vi "lwr_main.vi"(6 "inputValid":bool, 7 "readAddress":u16, 8 "endOfWave":bool, 9 "startRecording":bool, 10 "satCntP2":u16=12, 11 "input":cluster{"index":u16, "data":i16}) -> (0 "recordReady":bool, 2 "readData":i32, 3 "waveCount":u16)   [LabVIEW 2016]
uses:
  <vilib>/rvi/Emulation/niFpgaEmulationIsFPGAContextNoSignature.vi
  <vilib>/rvi/DataTransferAndStorage/Container/Common/niFpgaContainerGetUniqueNameForEmu.vi
  <vilib>/rvi/Memory/Memory_Emulation/niFpgaMemoryEmulationCacheClearOnFirstRun.vi
  <vilib>/rvi/Memory/Memory_Emulation/nirvimemoryEmulationManagerCache_MakeExclusive.vi
  <vilib>/rvi/Memory/Memory_Emulation/niFpgaMemoryEmulationValidateCache.vi
  <vilib>/rvi/Memory/Memory_Emulation/nirvimemoryEmulationManagerCache_InsertValue.vi
  <vilib>/Utility/error.llb/Clear Errors.vi
  <vilib>/rvi/Memory/Memory_Emulation/nirvimemoryEmulationManagerCache_ReleaseExclusive.vi
  <vilib>/rvi/Memory/Memory_Emulation/nirvimemoryEmulationManagerCache_GetValue.vi
  <vilib>/rvi/Memory/Memory_Emulation/nirvimemoryEmulationManagerCache_SetValue.vi
  <vilib>/rvi/Emulation/niFpgaProcessEmulError.vi
  <vilib>/rvi/Emulation/niFpgaSctlEmulationGetInTimedLoop.vi
  <vilib>/rvi/Memory/Memory_Emulation/nirvimemoryFastEmulation.vi
  <vilib>/rvi/Memory/Memory_Emulation/nirvimemoryEmulation.vi
  <vilib>/rvi/errors/nirviReportUnexpectedCaseInternalError (U32).vi
  <vilib>/rvi/DataTransferAndStorage/Container/XNode/niFpgaContainer.xnode
  <vilib>/rvi/DataTransferAndStorage/Register/Emulation/niFpgaRegisterEmulation.vi
  <instrlib>/_niInstr/Basic Elements/v1/FPGA/niInstr Basic Elements v1 FPGA.lvlib
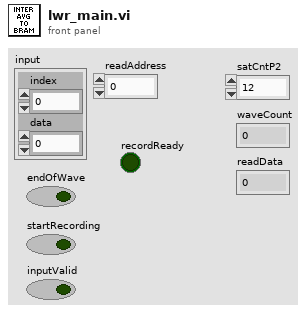
[diagram p1: front panel]
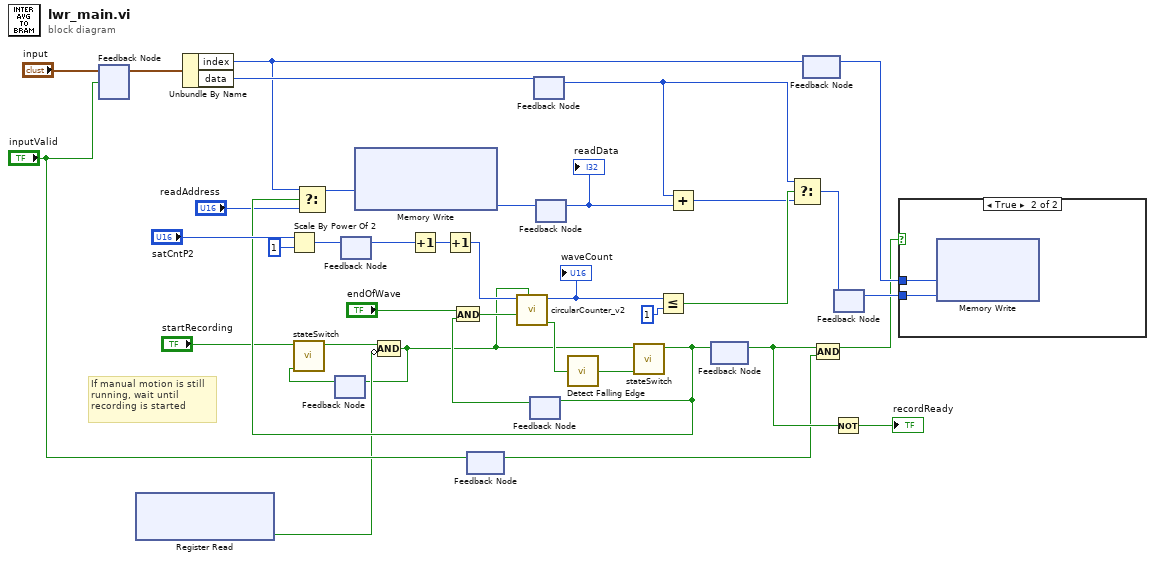
[diagram p0: block diagram]
diagram:
  # "If manual motion is still\nrunning, wait until \nrecording is started"
  n1 = feedback-in #1("input", "inputValid") -> ()
  n2 = feedback #1() -> (w12:cluster{"index":u16, "data":i16})  [unwired: 1 in]
  n3 = xnode ("Register Read")() -> ("Data"=w2:bool)  [unwired: 1 in, 1 out]
  n4 = Unbundle By Name(w12) -> ("index"=w14:u16, "data"=w38:i16)
  n5 = Scale By Power Of 2(n="satCntP2", x=u16 1) -> (x*2^n=w30:u16)
  n6 = feedback #2() -> (w3:bool)  [unwired: 1 in]
  n7 = call "stateSwitch.vi"("disable"=w3, "enable"="startRecording") -> ("state"=w4:bool)  [unwired: 9 in]
  n8 = feedback #3() -> (w34:u16)  [unwired: 1 in]
  n9 = feedback-in #3(w30) -> ()
  n10 = Compound Arithmetic op=AND(w4, invert w2) -> (w1:bool)
  n11 = feedback-in #2(w1) -> ()
  n12 = Increment(x=w34) -> (x+1=w18:u16)
  n13 = Increment(x=w18) -> (x+1=w22:u16)
  n14 = feedback-in #4("inputValid") -> ()
  n15 = feedback #4() -> (w9:bool)  [unwired: 1 in]
  n16 = feedback #5() -> (w24:bool)  [unwired: 1 in]
  n17 = And(x="endOfWave", y=w24) -> (x .and. y?=w37:bool)
  n18 = call "circularCounter_v2.vi"("reset"=w1, "doStep"=w37, "maxCount"=w22) -> ("maxReached"=w25:bool, "index"=w21:u16)  [unwired: 5 in, 2 out]
  "waveCount" <- w21
  n19 = feedback #6() -> (w16:i16)  [unwired: 1 in]
  n20 = feedback-in #6(w38) -> ()
  n21 = feedback #7() -> (w28:i32)  [unwired: 1 in]
  "readData" <- w28
  n22 = call <instrlib>:"Detect Falling Edge.vi"("signal"=w25) -> ("edge detected"=w19:bool)  [unwired: 14 in]
  n23 = call "stateSwitch.vi"("disable"=w19, "enable"=w1) -> ("state"=w7:bool)  [unwired: 9 in]
  n24 = Select(t=w14, s=w7, f="readAddress") -> (s? t:f=w8:u16)
  n25 = xnode ("Memory Write")("Address"=w8) -> ("Data"=w32:i32)  [unwired: 1 in, 1 out]
  n26 = feedback-in #5(w7) -> ()
  n27 = feedback-in #7(w32) -> ()
  n28 = Less Or Equal?(x=w21, y=u16 1) -> (x <= y?=w36:bool)
  n29 = Add(x=w16, y=w28) -> (x+y=w26:i32)
  n30 = feedback #8() -> (w23:bool)  [unwired: 1 in]
  n31 = feedback-in #8(w7) -> ()
  n32 = Select(t=w16, s=w36, f=w26) -> (s? t:f=w31:i32)
  n33 = feedback-in #9(w14) -> ()
  n34 = feedback #9() -> (w13:u16)  [unwired: 1 in]
  n35 = Compound Arithmetic op=AND(w23, w9) -> (w11:bool)
  n36 = Not(x=w23) -> (.not. x?=→"recordReady":bool)
  n37 = feedback #10() -> (w33:i32)  [unwired: 1 in]
  n38 = feedback-in #10(w31) -> ()
  n39 = case shown="True" w11 {
    tunnel: w33 -> [_ w40]
    tunnel: w13 -> [_ w39]
    frame False {
    }
    frame True {
      n40 = xnode ("Memory Write")("Address"=w39, "Data"=w40) -> ()  [unwired: 1 in, 1 out]
    }
  }
